vi "Convert Millimeters To Machine Units.vi"(9 "Distance (mm)":dbl, 10 "CMD LUT":variant, 11 "Axis No.":u8=1 min=1 max=4) -> (1 "Distance (MU)":u32 caption="Distance (Machine Units)")   [LabVIEW 2026, in "MicroPulse_Driver.lvlib"]
uses:
  MicroPulse_Driver.lvlib
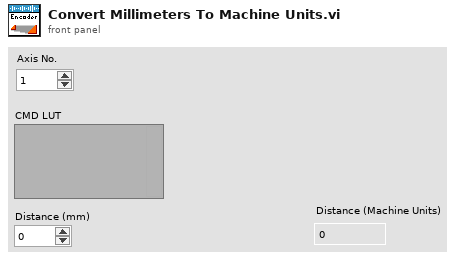
[diagram p1: front panel]
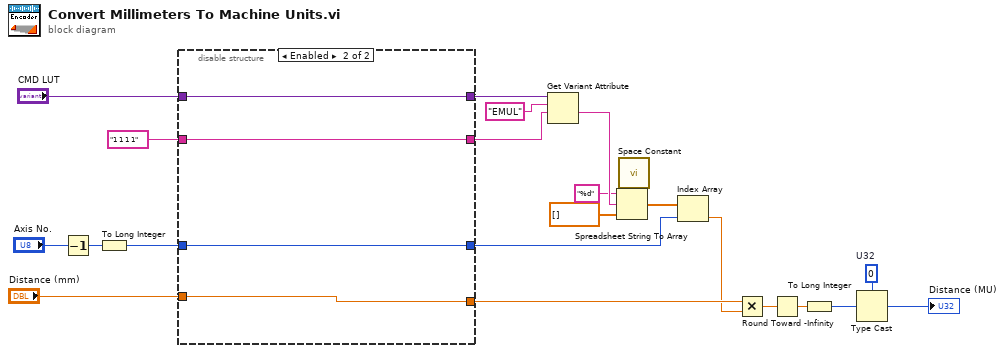
[diagram p0: block diagram]
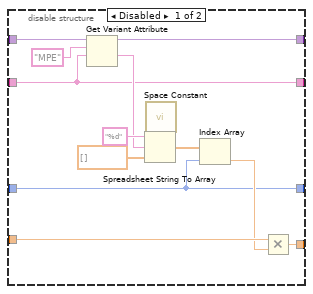
[diagram p2: hidden frame]
diagram:
  w2 = u32 0  # U32
  n1 = Decrement(x="Axis No.") -> (x-1=w8:u8)
  n2 = To Long Integer(number=w8) -> (32bit integer=w7:i32)
  n3 = disable-structure shown="Enabled" {
    disable-tunnel: [w24 w38] -> w20
    disable-tunnel: [w32 w39] -> w18
    disable-tunnel: "CMD LUT" -> [w30 w39]
    disable-tunnel: "Distance (mm)" -> [w27 w37]
    disable-tunnel: [w25 w37] -> w11
    disable-tunnel: w7 -> [w23 w36]
    disable-tunnel: "1 1 1 1" -> [w24 w38]
    disable-tunnel: [w23 w36] -> w5
    frame Disabled {
      n4 = Get Variant Attribute(Variant=w30, name="MPE", default value (empty Variant)=w24) -> (duplicate Variant=w32:variant, value=w33:string)  [unwired: 1 in, 2 out]
      n5 = call <vilib>:"Space Constant.vi"() -> ("String"=w35:string)
      n6 = Spreadsheet String To Array(delimiter (Tab)=w35, format string="%d", spreadsheet string=w33, array type (2D Dbl)=dbl[] []) -> (array=w28:dbl[])
      n7 = Index Array(array=w28, index=w23) -> (element=w26:dbl)
      n8 = Multiply(x=w27, y=w26) -> (x*y=w25:dbl)
    }
    frame Enabled {
    }
  }
  n9 = Get Variant Attribute(Variant=w18, name="EMUL", default value (empty Variant)=w20) -> (value=w22:string)  [unwired: 1 in, 3 out]
  n10 = call <vilib>:"Space Constant.vi"() -> ("String"=w16:string)
  n11 = Spreadsheet String To Array(delimiter (Tab)=w16, format string="%d", spreadsheet string=w22, array type (2D Dbl)=dbl[] []) -> (array=w13:dbl[])
  n12 = Index Array(array=w13, index=w5) -> (element=w10:dbl)
  n13 = Multiply(x=w11, y=w10) -> (x*y=w9:dbl)
  n14 = Round Toward -Infinity(1:w9) -> (0:w4:dbl)
  n15 = To Long Integer(number=w4) -> (32bit integer=w3:i32)
  n16 = Type Cast(type=w2, x=w3) -> (*(type *) &x=→"Distance (MU)":u32)
